vi "Single Example.vi"() -> ()   [LabVIEW 2020]
uses:
  <vilib>/NI/Modbus Library/API/Wrapper/Create Serial Master.vi
  <vilib>/NI/Modbus Library/API/Master/Modbus Master.lvclass
  <vilib>/NI/Modbus Library/API/Wrapper/API Main.lvlib
panel:
  in  "Direction Switch":bool
  in  "ON/OFF - Switch":bool
  in  "stop":bool
  in  "Vertical Frequencey Setting (Hz) - Manual":dbl caption="Vertical Frequencey Setting (Hz)" min=0.0 max=60.0 step=1.0
  in  "VISA resource name":refnum<visa-resource-name>
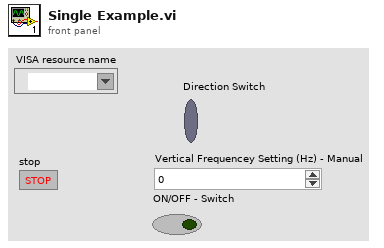
[diagram p1: front panel]
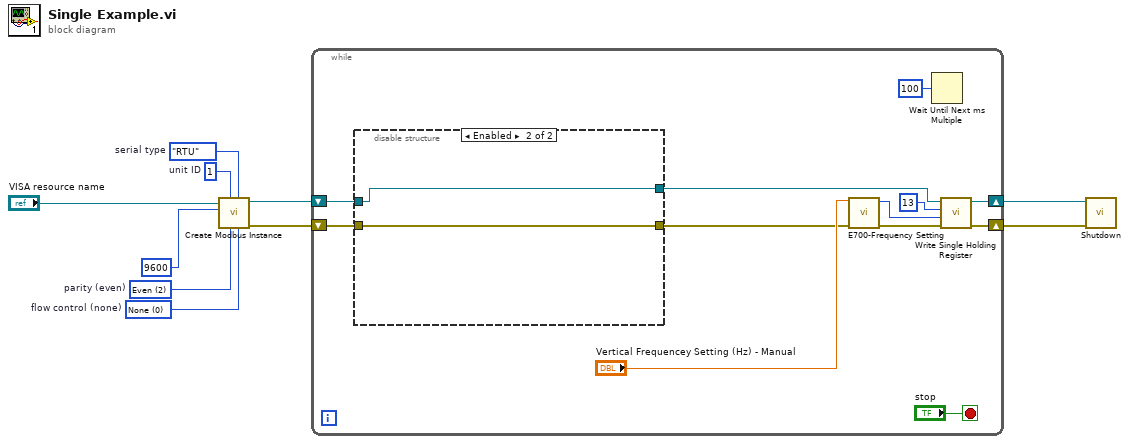
[diagram p0: block diagram]
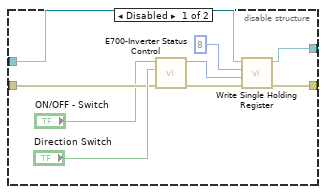
[diagram p2: hidden frame]
diagram:
  w10 = u16 0 items=["None", "XON/XOFF", "RTS/CTS", "XON/XOFF & RTS/CTS", "DTR/DSR", "XON/XOFF & DTR/DSR"]  # flow control (none)
  w8 = u16 2 items=["None", "Odd", "Even", "Mark", "Space"]  # parity (even)
  w9 = enum16{"RTU", "ASCII"}."RTU"  # serial type
  w7 = u8 1  # unit ID
  n1 = call-poly <vilib>:"Create Modbus Instance.vi"("flow control (none)"=w10, "serial type"=w9, "parity (even)"=w8, "unit ID"=w7, "baud rate"=u32 9600, "VISA resource name"="VISA resource name") -> ("error out"=w1:errorcluster, "serial master instance"=w4:refnum<class "Modbus Master.lvclass">)  [unwired: 4 in]
  n2 = while {
    shift-right: [w18] -> w3
    shift-left: w1 -> [w14]
    shift-right: [w17] -> w2
    shift-left: w4 -> [w13]
    stop <- "stop" stop-if-true
    n3 = disable-structure shown="Enabled" {
      disable-tunnel: w14 -> [w26 w32]
      disable-tunnel: w13 -> [w31 w33]
      disable-tunnel: [w30 w33] -> w12
      disable-tunnel: [w28 w32] -> w11
      frame Disabled {
        n4 = call "E700-Inverter Status Control.vi"("error in (no error)"=w26, "Direction Switch"="Direction Switch", "ON/OFF - Switch"="ON/OFF - Switch") -> ("error out"=w25:errorcluster, "Send Value"=w23:u16)  [unwired: 7 in]
        n5 = call-dynamic "Write Single Holding Register.vi"("error in"=w25, "register to write"=w23, "address"=u16 8, "Modbus master in"=w31) -> ("error out"=w28:errorcluster, "Modbus master out"=w30:refnum<class "Modbus Master.lvclass">)  [unwired: 6 in]
      }
      frame Enabled {
      }
    }
    n6 = call "E700-Frequency Setting.vi"("error in (no error)"=w11, "Frequencey Setting (Hz)"="Vertical Frequencey Setting (Hz) - Manual") -> ("error out"=w21:errorcluster, "Set Value"=w20:u16)  [unwired: 8 in]
    n7 = Wait Until Next ms Multiple(millisecond multiple=u32 100) -> ()  [unwired: 1 out]
    n8 = call-dynamic "Write Single Holding Register.vi"("error in"=w21, "register to write"=w20, "address"=u16 13, "Modbus master in"=w12) -> ("error out"=w18:errorcluster, "Modbus master out"=w17:refnum<class "Modbus Master.lvclass">)  [unwired: 6 in]
  }
  n9 = call-dynamic "Shutdown.vi"("error in"=w3, "Modbus master in"=w2) -> ()  [unwired: 9 in, 1 out]
